vi "Oscop Read Averaging.vi"(7 "Measurement (0: Vpp)":u16, 8 "error in (no error)":errorcluster, 9 "Source (1: Channel 1)":u16, 10 "Numeric in":i32, 11 "VISA Refnum in":refnum<visa-resource-name>) -> (0 "error out":errorcluster, 2 "Numeric out":dbl, 3 "VISA Refnum out":refnum<visa-resource-name>)   [LabVIEW 2021]
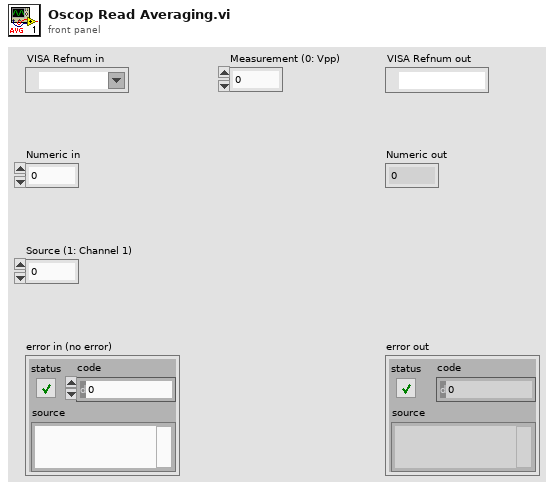
[diagram p1: front panel]
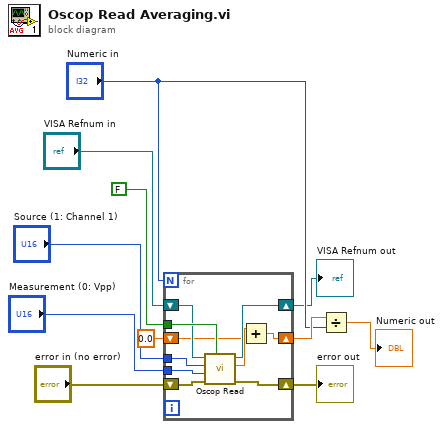
[diagram p0: block diagram]
diagram:
  n1 = for {
    N: "Numeric in" -> [_]
    tunnel: FALSE ("Perform Auto Setup") -> [w21]
    tunnel: "Measurement (0: Vpp)" -> [w16]
    tunnel: "Source (1: Channel 1)" -> [w15]
    shift-right: [w20] -> w3
    shift-left: "error in (no error)" -> [w19]
    shift-right: [w17] -> w6
    shift-left: "VISA Refnum in" -> [w18]
    shift-right: [w13] -> w11
    shift-left: 0.0 -> [w12]
    n2 = call "Oscop Read.vi"("Perform Auto Setup"=w21, "error in (no error)"=w19, "Measurement (0: Vpp)"=w16, "Source (1: Channel 1)"=w15, "VISA resource name"=w18) -> ("error out"=w20:errorcluster, "Value"=w14:dbl, "VISA resource name out"=w17:refnum<visa-resource-name>)  [unwired: 4 in]
    n3 = Add(x=w14, y=w12) -> (x+y=w13:dbl)
  }
  "VISA Refnum out" <- w6
  "error out" <- w3
  n4 = Divide(x=w11, y="Numeric in") -> (x/y=→"Numeric out":dbl)
